vi "Autonomous Independent.vi"() -> ()   [LabVIEW 2012]
doc: "This VI is called when autonomous begins, and will automatically be terminated when autonomous ends. You can carry out timed or sensor driven robot movement independently without needing to return to the caller."
uses:
  <vilib>/Rock Robotics/WPI/SafetyOutput/WPI_SafetyOutputConfigMenu.ctl
  Robot Global Data.vi
  Autonomous Global Data.vi
  <vilib>/Rock Robotics/WPI/RobotDrive/WPI_RobotDriveGetSetRefNum.vi
  <vilib>/Rock Robotics/WPI/RobotDrive/WPI_RobotDriveMecanumDrive_Cartesian.vi
  <vilib>/Rock Robotics/WPI/Joystick/WPI_JoystickGetSetRefNum.vi
  <vilib>/Rock Robotics/WPI/RobotDrive/WPI_RobotDriveArcadeDrive.vi
panel:
  in  "time":dbl
  in  "File Name With Extension 3":string="test1.cat"
  in  "File Name With Extension 2":string="test1.cat"
  in  "File Name With Extension 1":string="test1.cat"
  out "Autonomous Mode":u16(ring) items=["None", "Scripted", "Hybrided"]
  out "error out":errorcluster
  in  "File Name With Extension 0":string="test1.cat"
  out "File Status":string
  out "Lines":string[](array[string])
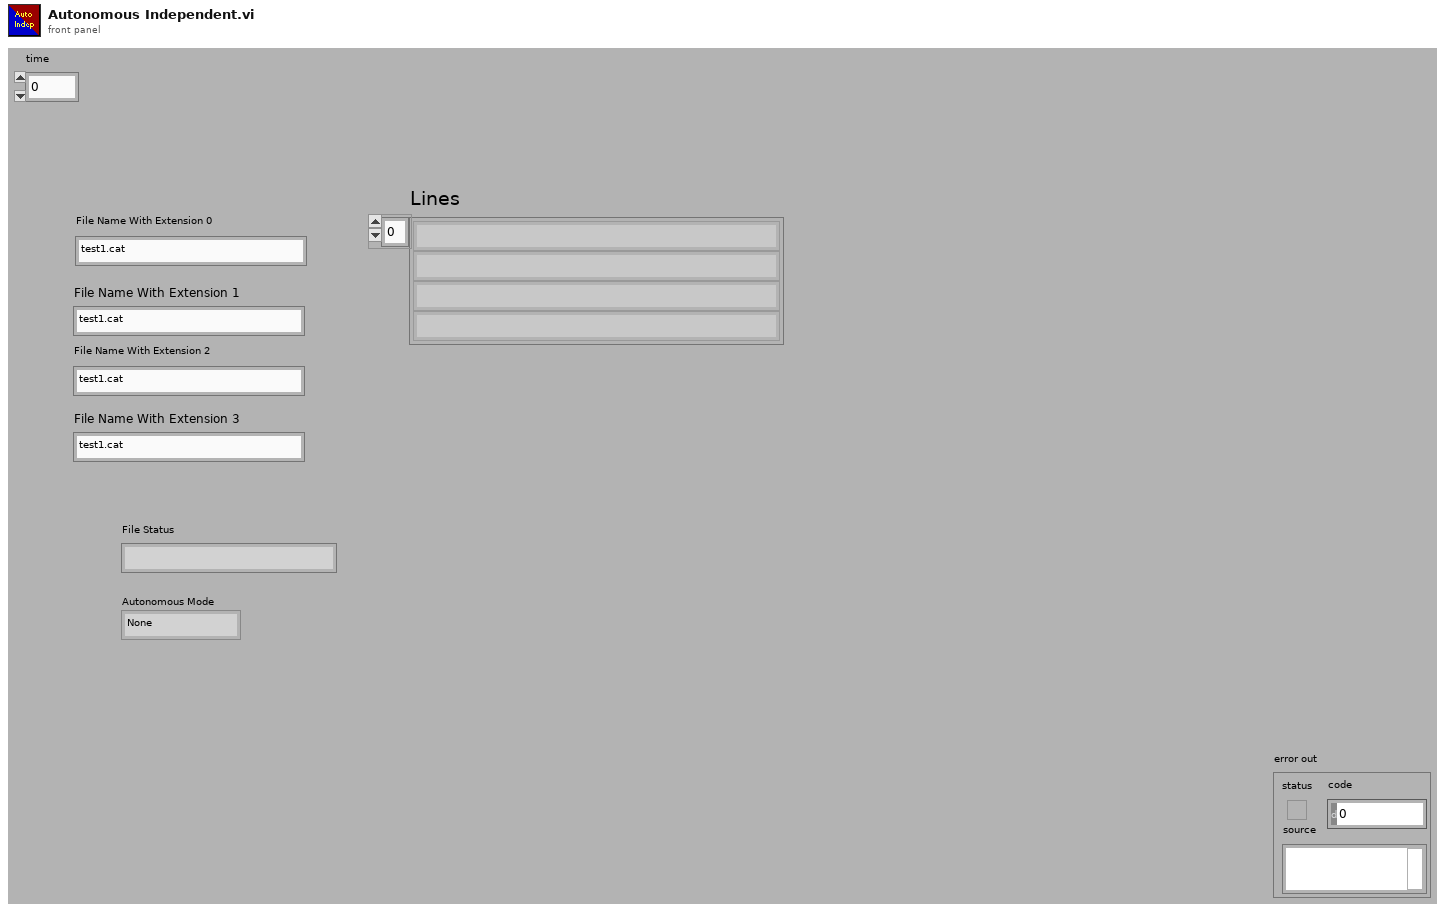
[diagram p1: front panel]
types:
  T1 = typedef "WPI_JoystickDevRef.ctl" = cluster{"Device":T2}
  T2 = typedef "WPI_JoystickDeviceEnum.ctl" = enum16{"USB 1", "USB 2", "USB 3", "USB 4", "Kinect 1", "Kinect 2"}
  T3 = cluster{"axis 1 (x)":dbl, "axis 2 (y)":dbl, "axis 3 (throttle)":dbl, "axis 4":dbl, "axis 5":dbl, "axis 6":dbl}
  T4 = typedef "WPI_SafetyOutputConfigMenu.ctl" = enum16{"Enable", "Disable"}
  T5 = typedef "WPI_RobotDriveDevRef.ctl" = cluster{"DevStatus":errorcluster, "Motors[]":T6[], "Square Inputs":bool, "Max Output":dbl, "Isochronous":bool}
  T6 = typedef "WPI_MotorControlDeviceRef.ctl" = cluster{"DeviceStatus":errorcluster, "Type":enum16{"PWM", "CAN"}, "PWM":cluster{"Digital Module":T7, "PWM Channel":T8, "DeadBand":T9}, "CAN":cluster{"Device Number":u8, "Control Mode":T10, "Semaphore":T11, "Max Vout":dbl}, "Invert":bool, "TransformRef":T12, "InvTransformRef":T12}
  T7 = typedef "FPGA_TypedefDigitalModule.ctl" = enum16{"Digital Module 1", "Digital Module 2"}
  T8 = typedef "FPGA_DIOPWMChannel.ctl" = enum8{"PWM 1", "PWM 2", "PWM 3", "PWM 4", "PWM 5", "PWM 6", "PWM 7", "PWM 8", "PWM 9", "PWM 10", "Invalid"}
  T9 = typedef "WPI_PWMDeadband.ctl" = cluster{"Name":string, "maxPositivePwm":i32, "minPositivePwm":i32, "centerPwm":i32, "maxNegativePwm":i32, "minNegativePwm":i32, "angularRange":u16}
  T10 = typedef "WPI_CANJaguar_ControlMode.ctl" = enum8{"Percent VBus", "Current", "Speed", "Position", "Voltage"}
  T11 = typedef "Semaphore RefNum" = refnum<k1>
  T12 = typedef "WPI_PWMTransform_ConPane.ctl" = refnum<vi>
  T13 = cluster{"RightAxis":dbl, "LeftAxis":dbl, "RightHead":bool, "Left Head":bool, "Left Leg Out":bool, "Left Leg Forward":bool, "Left Leg Back":bool, "Right Leg Out":bool, "Right Leg Forward":bool, "Right Leg Back":bool}
  T14 = cluster{"Position":cluster{"X":dbl, "Y":dbl}, "Distance (ft)":dbl}[]
  T15 = cluster{"Position":cluster{"X":dbl, "Y":dbl}, "Distance (ft)":dbl}
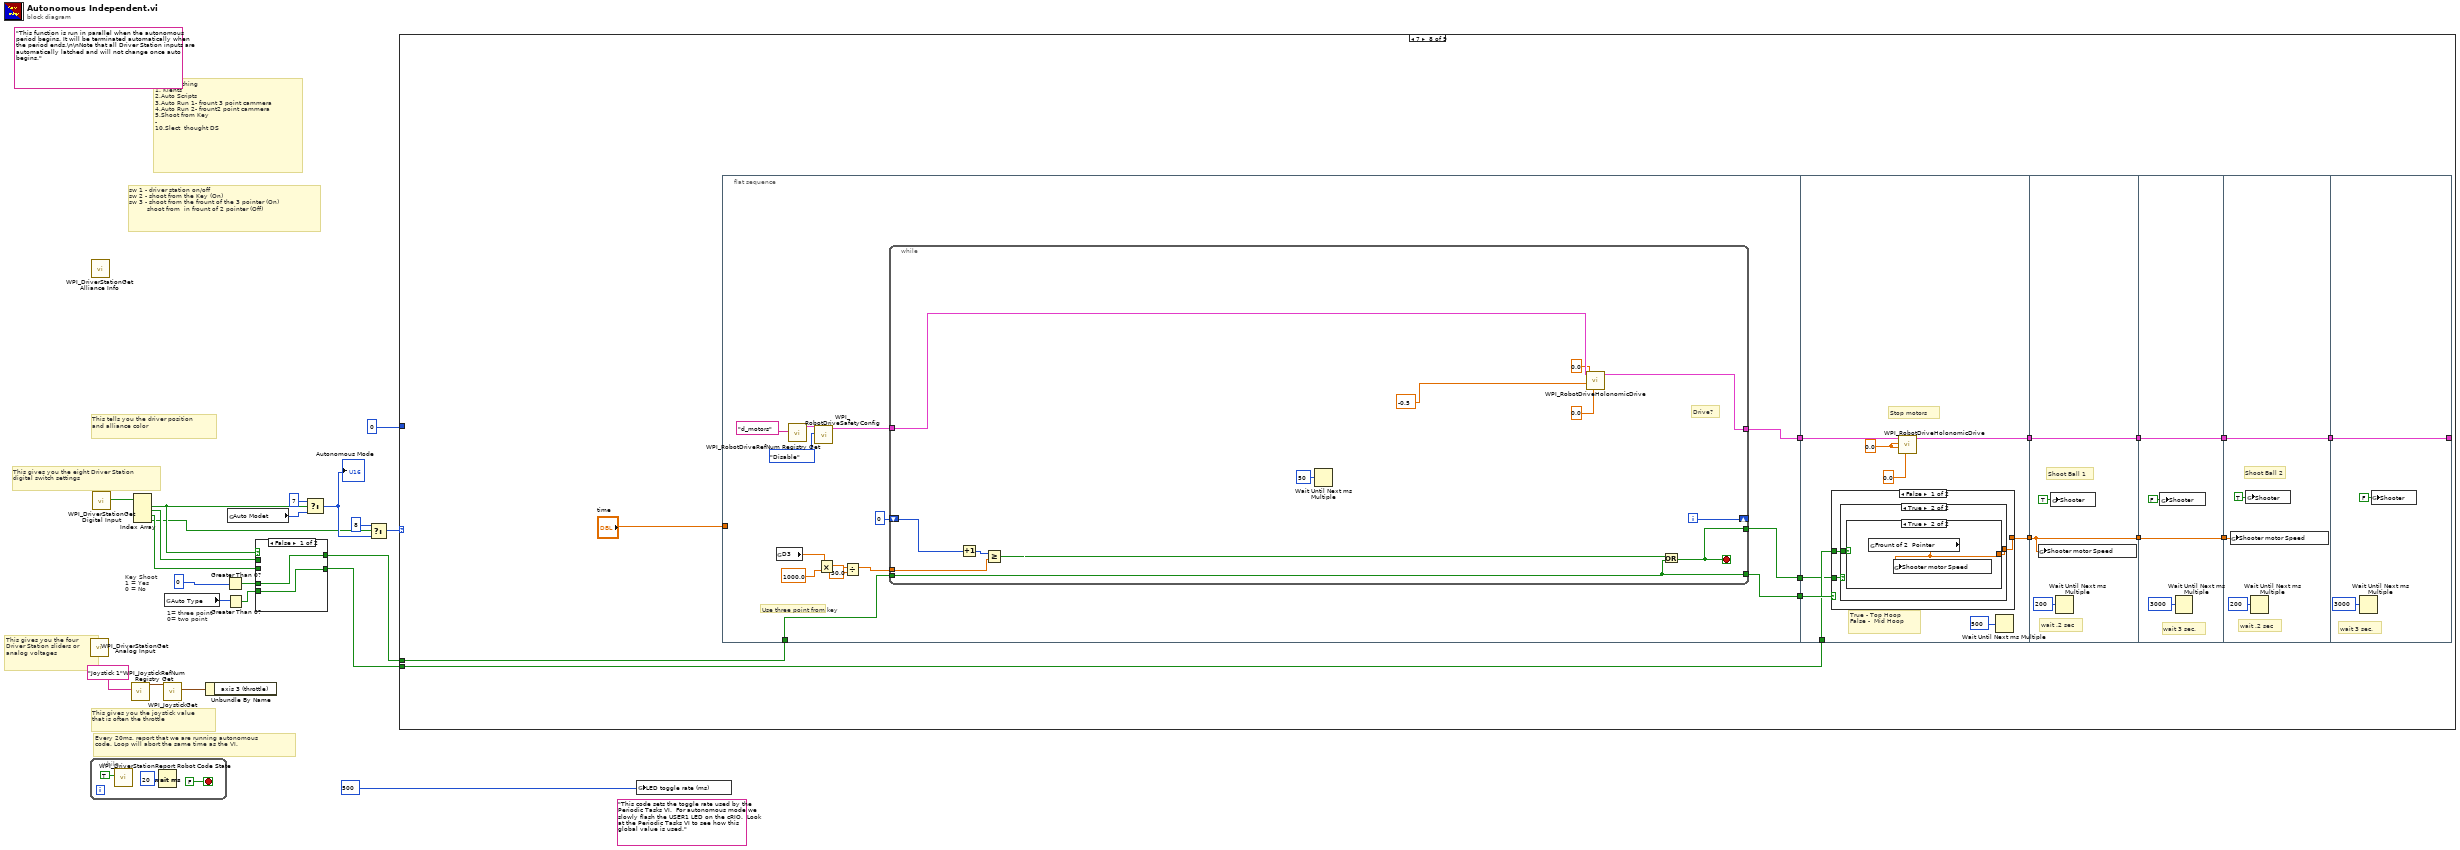
[diagram p0: block diagram]
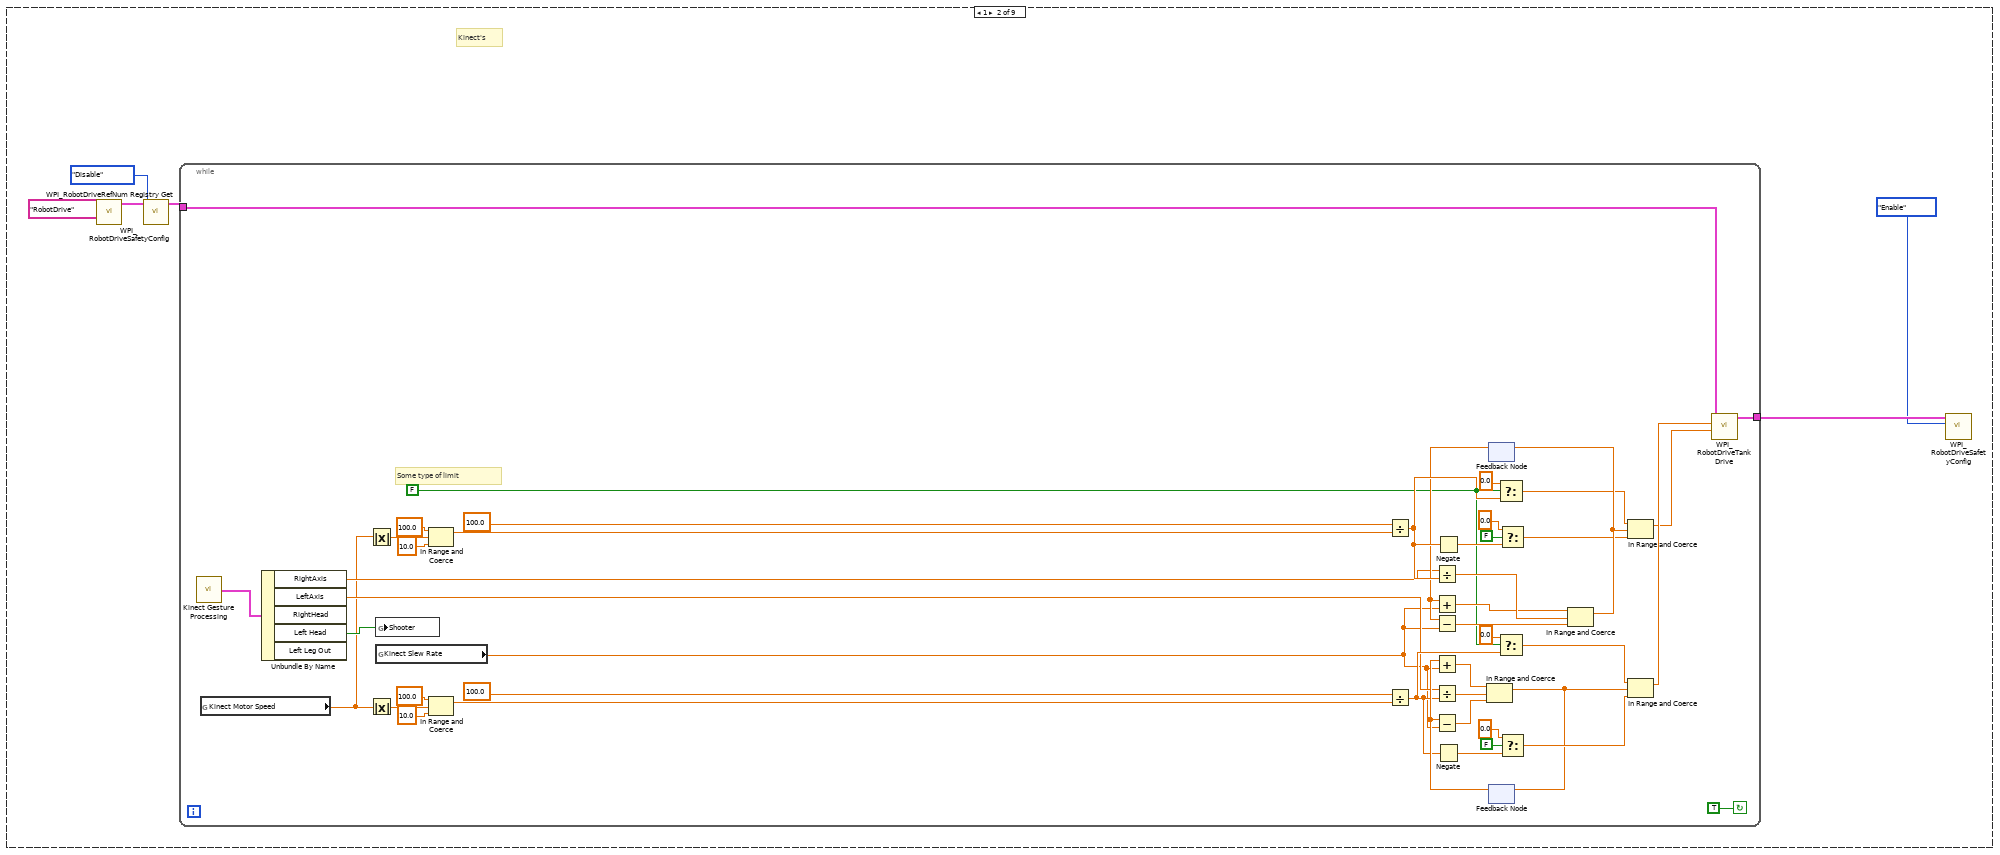
[diagram p4: hidden frame]
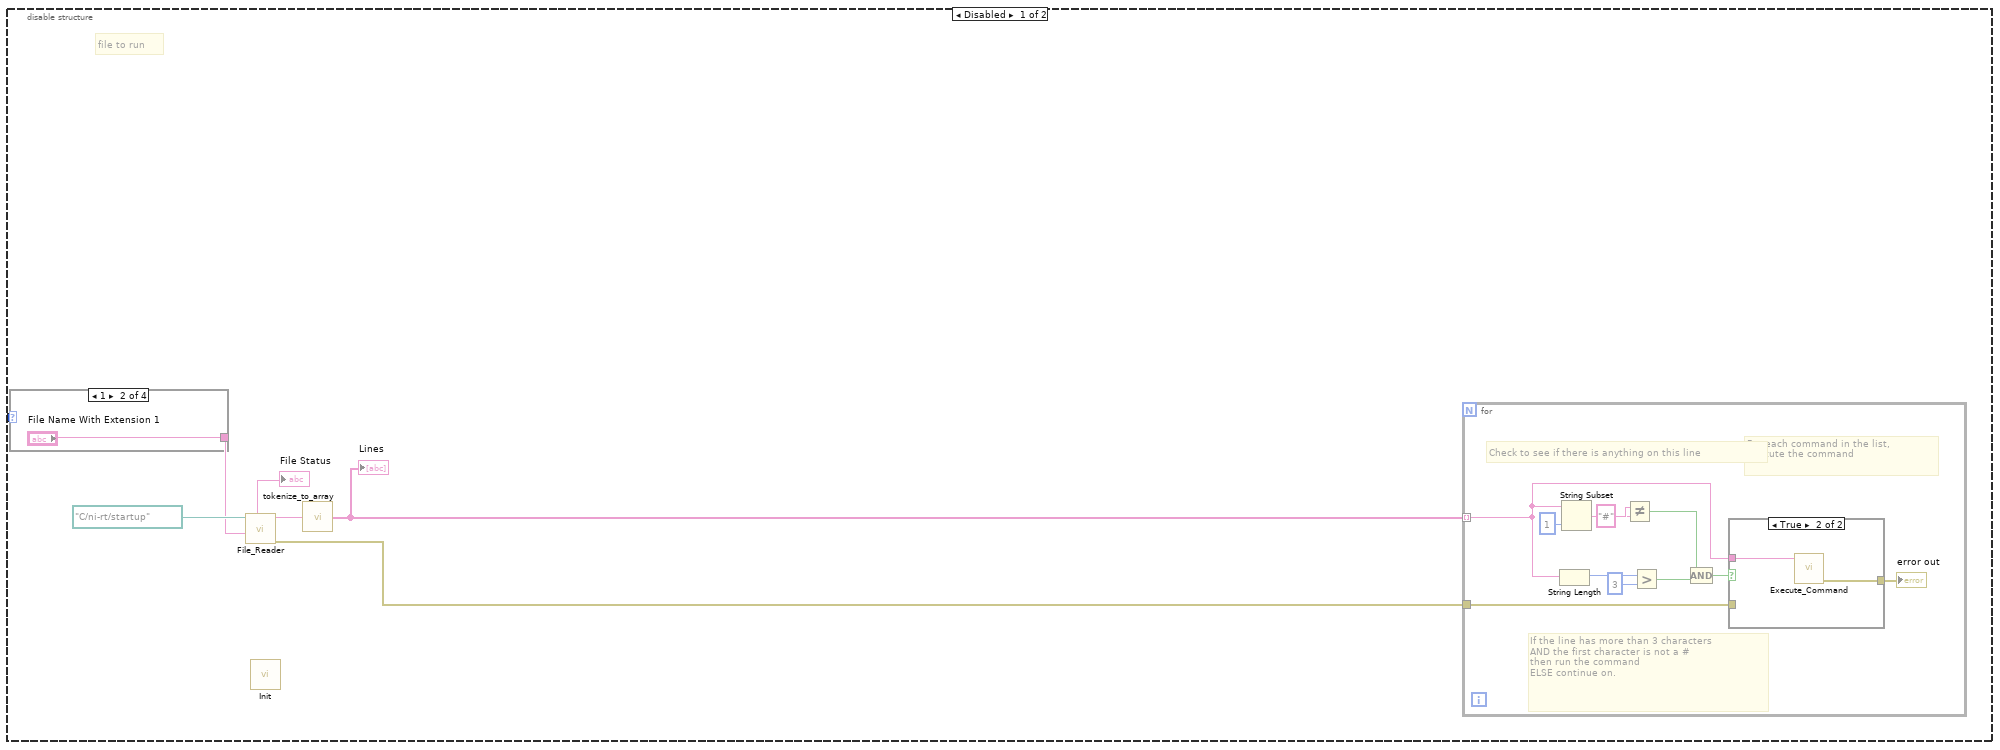
[diagram p6: hidden frame]
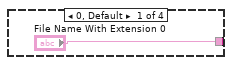
[diagram p7: hidden frame]
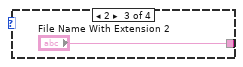
[diagram p8: hidden frame]
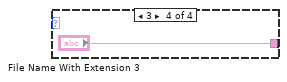
[diagram p9: hidden frame]
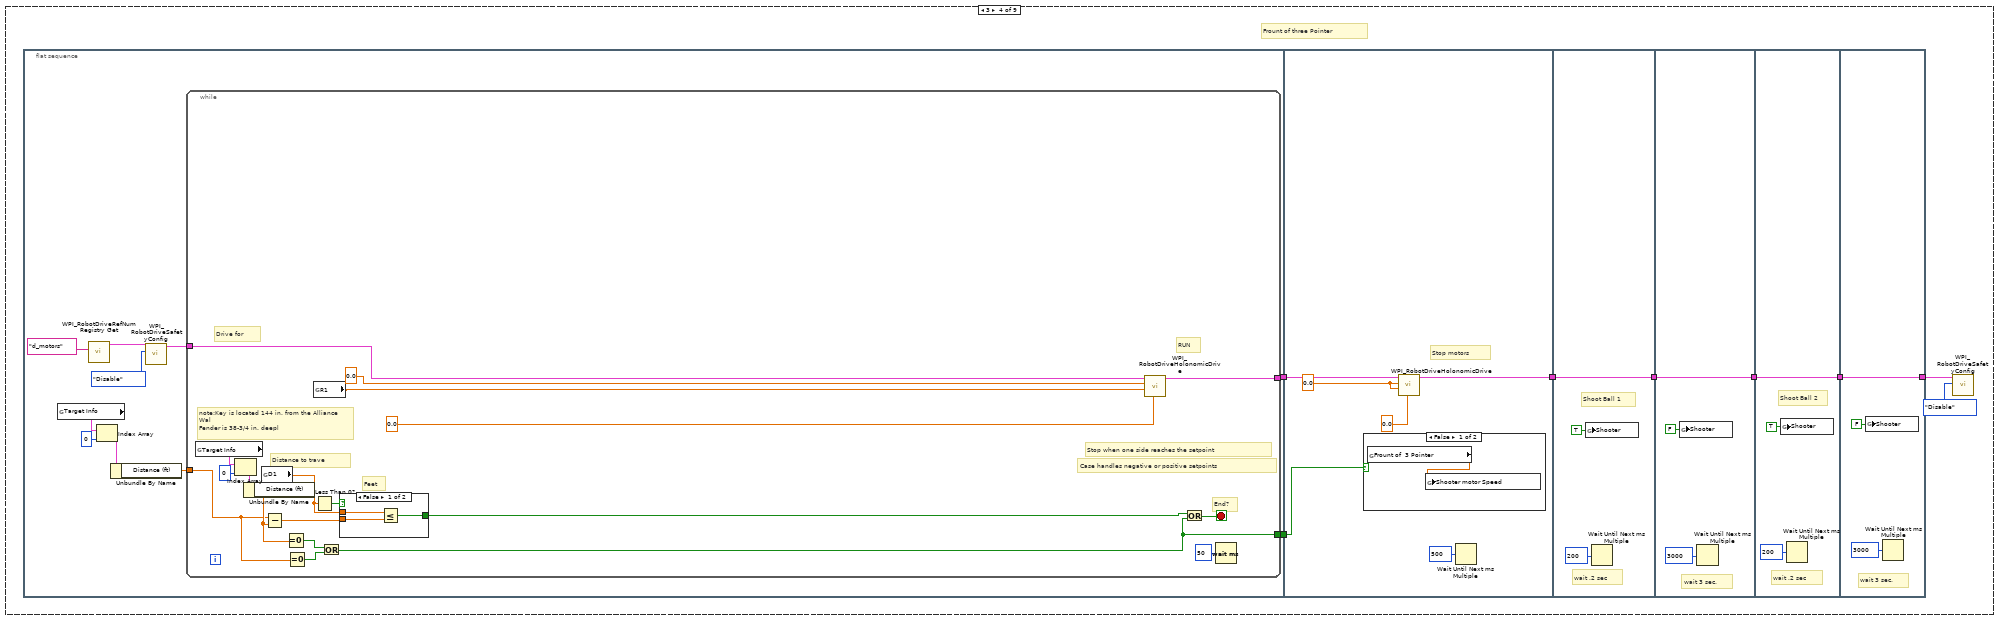
[diagram p11: hidden frame]
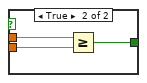
[diagram p12: hidden frame]
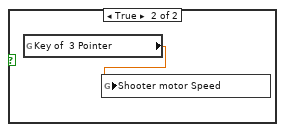
[diagram p13: hidden frame]
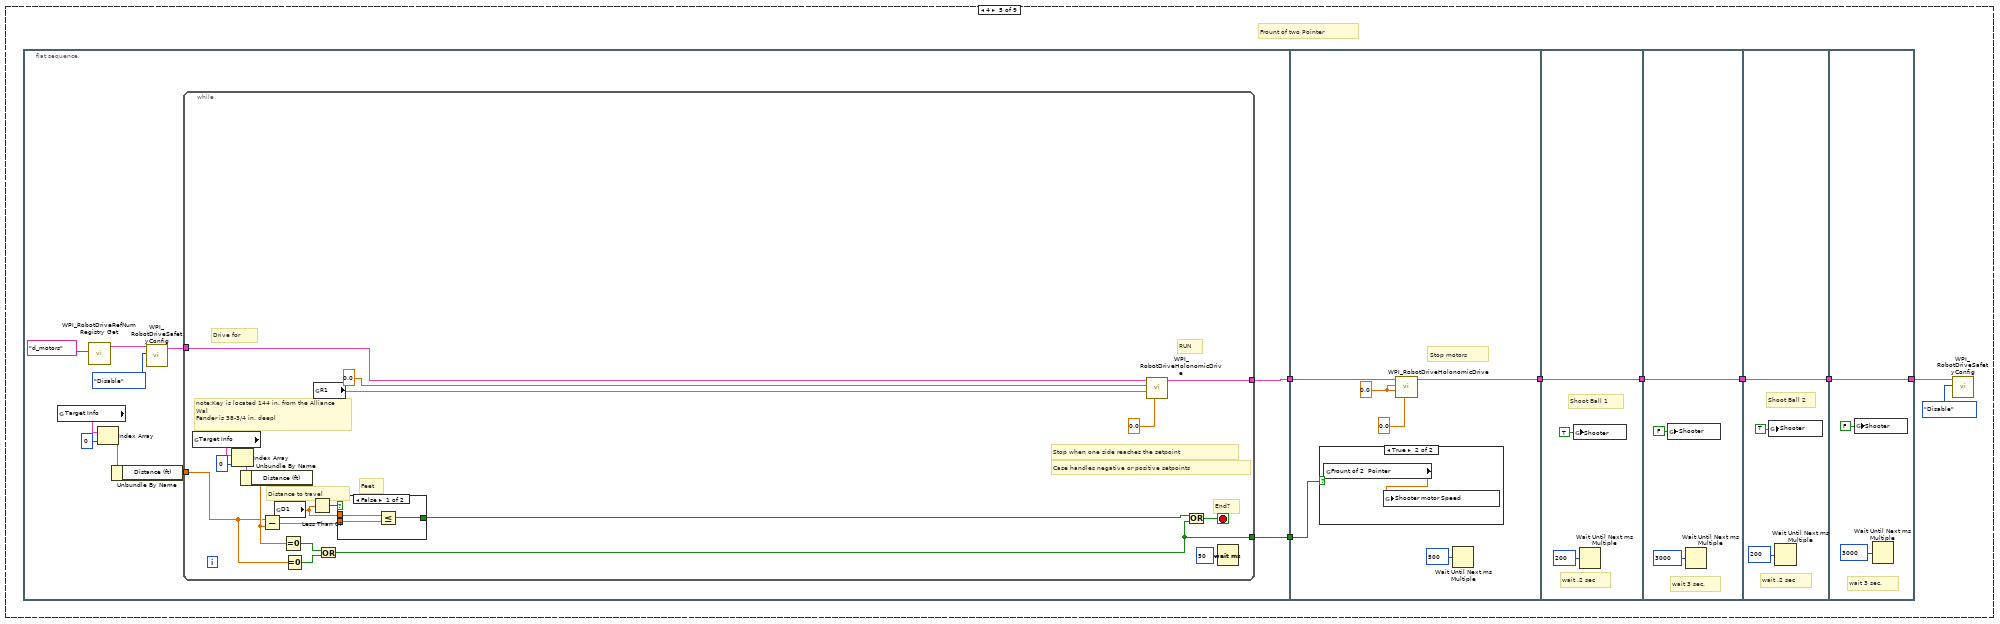
[diagram p14: hidden frame]
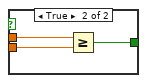
[diagram p15: hidden frame]
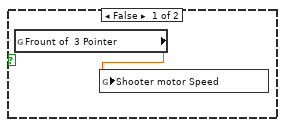
[diagram p16: hidden frame]
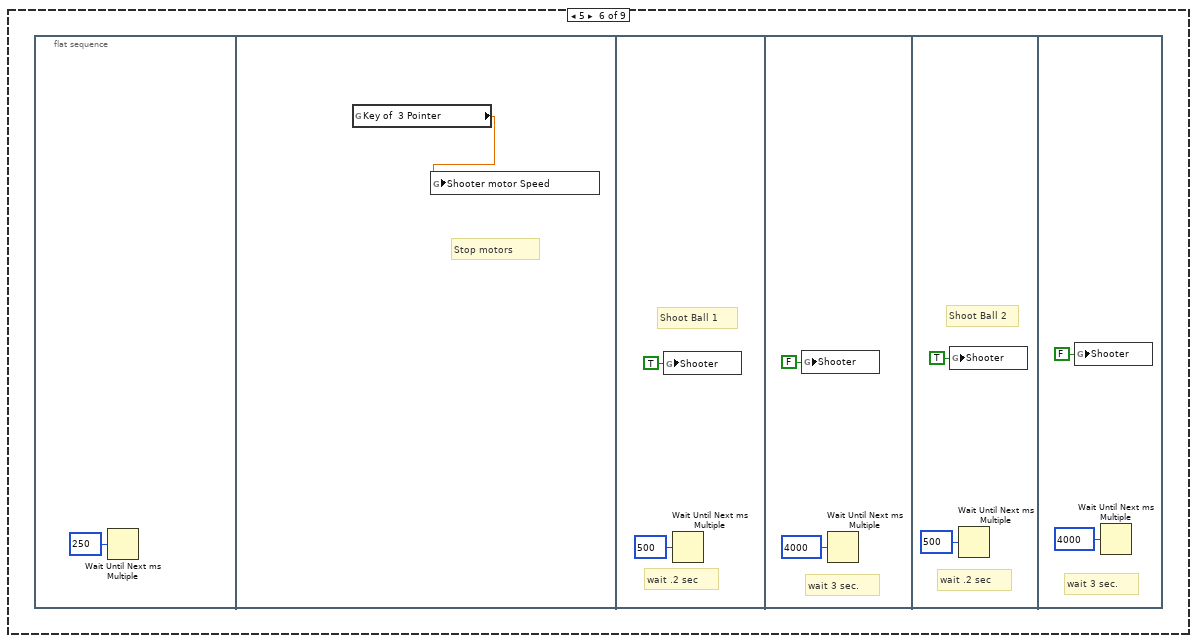
[diagram p17: hidden frame]
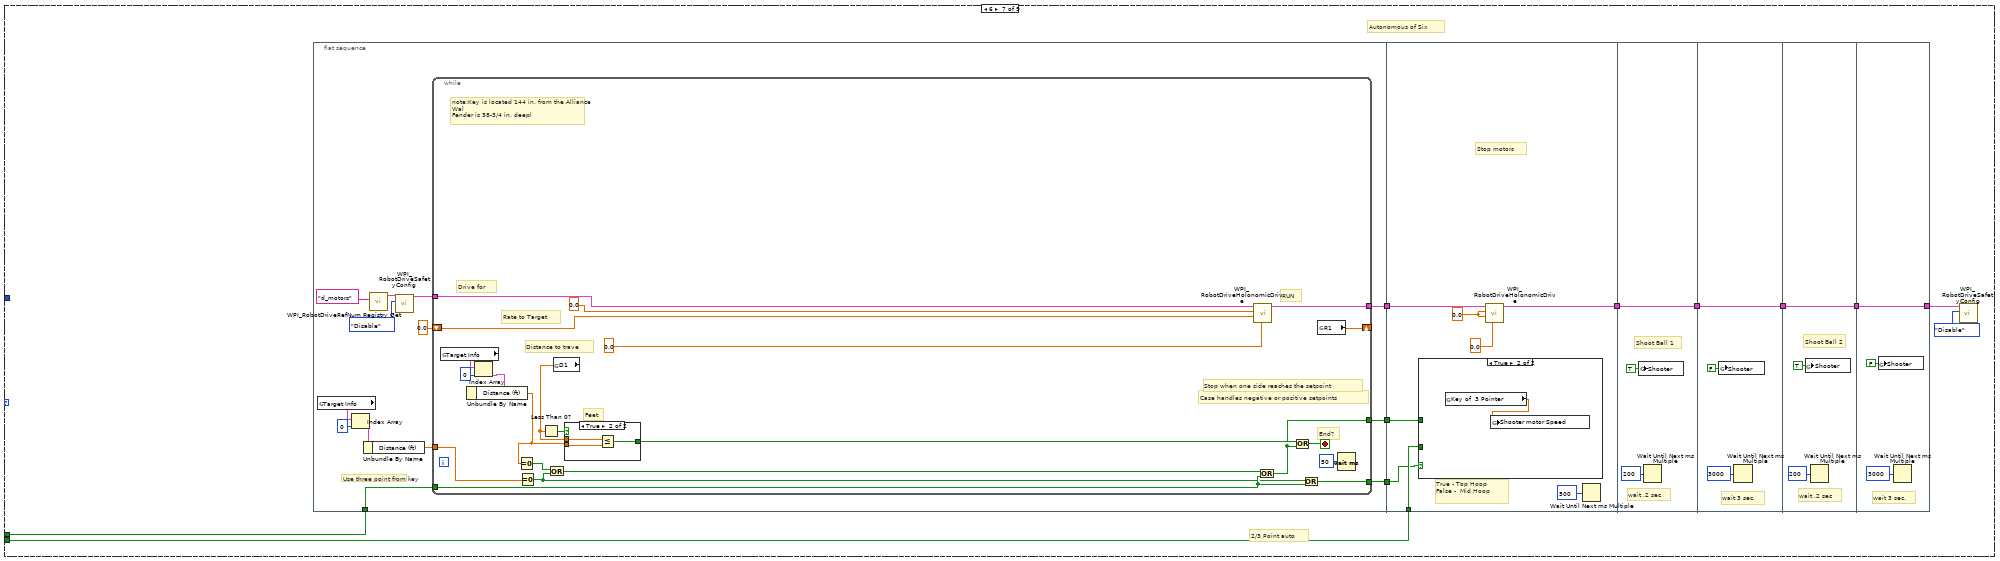
[diagram p18: hidden frame]
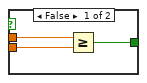
[diagram p19: hidden frame]
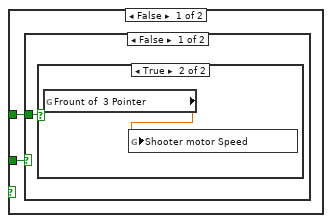
[diagram p20: hidden frame]
diagram:
  (unwired) "This code sets the toggle rate used by the Periodic Tasks VI.  For autonomous mode we slowly flash the USER1 LED on the cRIO.  Look at the Periodic Tasks VI to see how this global value is used."
  (unwired) "This function is run in parallel when the autonomous period begins. It will be terminated automatically when the period ends.\n\nNote that all Driver Station inputs are automatically latched and will not change once auto begins."
  # "Key Shoot\n1 = Yes\n0 = No"
  # "sw 1 - driver station on/off\nsw 2 - shoot from the Key (On)\nsw 3 - shoot from the frount of the 3 pointer (On)\n         shoot from  in frount of 2 pointer (Off)"
  # "1= three point\n0= two point"
  # "0. Do nothing\n1. Kients\n2.Auto Scripts\n3.Auto Run 1- frount 3 point cammera\n4.Auto Run 2- frount2 point cammera\n5.Shoot from Key\n-\n10.Slect  thought DS"
  # "Every 20ms, report that we are running autonomous\ncode. Loop will abort the same time as the VI."
  # "This gives you the joystick value\nthat is often the throttle"
  # "This tells you the driver position\nand alliance color"
  # "This gives you the eight Driver Station\ndigital switch settings"
  # "This gives you the four\nDriver Station sliders or\nanalog voltages"
  n1 = call <vilib>:"WPI_DriverStationGet Analog Input.vi"() -> ()  [unwired: 12 out]
  n2 = while {
    stop <- FALSE stop-if-true
    n3 = call <vilib>:"WPI_DriverStationReport Robot Code State.vi"("Autonomous"=TRUE) -> ()  [unwired: 10 in, 1 out]
    n4 = Wait (ms)(milliseconds to wait=u32 20) -> ()  [unwired: 1 out]
  }
  n5 = call <vilib>:"WPI_DriverStationGet Alliance Info.vi"() -> ()  [unwired: 12 out]
  n6 = call <vilib>:"WPI_DriverStationGet Digital Input.vi"() -> ("Driver Station Digital Input (1-8)"=w21:bool[])  [unwired: 11 out]
  n7 = call <vilib>:"WPI_JoystickRefNum Registry Get.vi"("refnum name"="Joystick 1") -> ("JoystickDevRef"=w18:T1)  [unwired: 1 in, 9 out]
  n8 = Index Array(array=w21) -> (element #1=w8:bool, element #2=w7:bool, element #3=w6:bool, element #4=w4:bool)  [unwired: 4 in]
  n9 = call <vilib>:"WPI_JoystickGet.vi"("JoystickDevRef"=w18) -> ("Axes"=w19:T3)  [unwired: 1 in, 5 out]
  n10 = global read "Autonomous Global Data.vi" "Auto Type"() -> (w14:u16)
  n11 = Unbundle By Name(w19) -> ()  [unwired: 1 out]
  n12 = Greater Than 0?(x=u16 0 ("t")) -> (x > 0?=w13:bool)
  n13 = Greater Than 0?(x=w14) -> (x > 0?=w12:bool)
  n14 = global read "Autonomous Global Data.vi" "Auto Modet"() -> (w10:u16)
  n15 = case shown="False" w8 {
    tunnel: w7 -> [_ w28]
    tunnel: w6 -> [_ w27]
    tunnel: [w26 w28] -> w16
    tunnel: [w25 w27] -> w15
    tunnel: w13 -> [w26 _]
    tunnel: w12 -> [w25 _]
    frame False {
    }
    frame True {
    }
  }
  n16 = Select(t=u16 7, s=w8, f=w10) -> (s? t:f=w11:u16)
  "Autonomous Mode" <- w11
  n17 = Select(t=u16 8, s=w4, f=w11) -> (s? t:f=w5:u16)
  n18 = case shown="7" w5 {
    tunnel: 0 -> [_ _ w81 _ _ _ _ _ _]
    tunnel: w15 -> [_ _ _ _ _ _ w245 w330 _]
    tunnel: w16 -> [_ _ _ _ _ _ w244 w331 _]
    frame 0, Default {
      # "Do nothing"
    }
    frame 1 {
      # "Kinect's"
      n19 = call <vilib>:"WPI_RobotDriveRefNum Registry Get.vi"("refnum name"="RobotDrive") -> ("RobotDriveDevRef"=w33:T5)  [unwired: 9 in, 1 out]
      n20 = call <vilib>:"WPI_RobotDriveSafetyConfig.vi"("mode"=WPI_SafetyOutputConfigMenu."Disable", "RobotDriveDevRef"=w33) -> ("RobotDriveDevRef"=w32:T5)  [unwired: 8 in, 1 out]
      n21 = while {
        tunnel: w32 -> [w79]
        tunnel: [w35] -> w30
        stop <- TRUE continue-if-true
        w36 = FALSE
        # "Some type of limit"
        n22 = call "Kinect Gesture Processing.vi"() -> ("Joystick Data"=w80:T13)  [unwired: 1 in]
        n23 = global read "Robot Global Data.vi" "Kinect Motor Speed"() -> (w40:dbl)
        n24 = Unbundle By Name(w80) -> ("RightAxis"=w42:dbl, "LeftAxis"=w41:dbl, "Left Head"=w77:bool)  [unwired: 2 out]
        n25 = Absolute Value(x=w40) -> (abs(x)=w50:dbl)
        n26 = Absolute Value(x=w40) -> (abs(x)=w67:dbl)
        n27 = global write "Robot Global Data.vi" "Shooter"(w77) -> ()
        n28 = global read "Robot Global Data.vi" "Kinect Slew Rate"() -> (w39:dbl)
        n29 = In Range and Coerce(upper limit=100.0, x=w50, lower limit=10.0) -> (coerced(x)=w53:dbl)  [unwired: 1 out]
        n30 = In Range and Coerce(upper limit=100.0, x=w67, lower limit=10.0) -> (coerced(x)=w64:dbl)  [unwired: 1 out]
        n31 = Divide(x=100.0, y=w53) -> (x/y=w56:dbl)
        n32 = Divide(x=100.0, y=w64) -> (x/y=w61:dbl)
        n33 = Divide(x=w42, y=w56) -> (x/y=w54:dbl)
        n34 = Divide(x=w41, y=w61) -> (x/y=w63:dbl)
        n35 = Negate(x=w56) -> (-x=w57:dbl)
        n36 = Negate(x=w61) -> (-x=w60:dbl)
        n37 = feedback #1() -> (w47:dbl)  [unwired: 1 in]
        n38 = Add(x=w47, y=w39) -> (x+y=w49:dbl)
        n39 = Subtract(x=w47, y=w39) -> (x-y=w48:dbl)
        n40 = feedback #2() -> (w70:dbl)  [unwired: 1 in]
        n41 = Add(x=w70, y=w39) -> (x+y=w68:dbl)
        n42 = Subtract(x=w70, y=w39) -> (x-y=w69:dbl)
        n43 = In Range and Coerce(upper limit=w68, x=w63, lower limit=w69) -> (coerced(x)=w62:dbl)  [unwired: 1 out]
        n44 = feedback-in #2(w62) -> ()
        n45 = Select(t=0.0, s=w36, f=w56) -> (s? t:f=w43:dbl)
        n46 = Select(t=0.0, s=w36, f=w61) -> (s? t:f=w74:dbl)
        n47 = Select(t=0.0, s=FALSE, f=w57) -> (s? t:f=w44:dbl)
        n48 = Select(t=0.0, s=FALSE, f=w60) -> (s? t:f=w73:dbl)
        n49 = In Range and Coerce(upper limit=w49, x=w54, lower limit=w48) -> (coerced(x)=w55:dbl)  [unwired: 1 out]
        n50 = feedback-in #1(w55) -> ()
        n51 = In Range and Coerce(upper limit=w43, x=w55, lower limit=w44) -> (coerced(x)=w37:dbl)  [unwired: 1 out]
        n52 = In Range and Coerce(upper limit=w74, x=w62, lower limit=w73) -> (coerced(x)=w38:dbl)  [unwired: 1 out]
        n53 = call <vilib>:"WPI_RobotDriveTankDrive.vi"("Right axis value"=w37, "Left axis value"=w38, "RobotDriveDevRef"=w79) -> ("RobotDriveDevRef"=w35:T5)  [unwired: 6 in, 2 out]
      }
      n54 = call <vilib>:"WPI_RobotDriveSafetyConfig.vi"("mode"=WPI_SafetyOutputConfigMenu."Enable", "RobotDriveDevRef"=w30) -> ()  [unwired: 8 in, 2 out]
    }
    frame 2 {
      n55 = disable-structure shown="Enabled" {
        disable-tunnel: w81 -> [w85 _]
        frame Disabled {
          # "file to run"
          n56 = case shown="1" w85 {
            tunnel: ["File Name With Extension 0" "File Name With Extension 1" "File Name With Extension 2" "File Name With Extension 3"] -> w82
            frame 0, Default {
            }
            frame 1 {
            }
            frame 2 {
            }
            frame 3 {
            }
          }
          n57 = call "File_Reader.vi"("File Name With Extension"=w82, "Path"=path "C:/ni-rt/startup") -> ("error out"=w86:errorcluster, "File Contents"=w88:string, "File status"=→"File Status":string)  [unwired: 2 in, 3 out]
          n58 = call "Init.vi"() -> ()  [unwired: 12 in]
          n59 = call "tokenize_to_array.vi"("File Contents"=w88) -> ("Lines"=w87:string[])
          "Lines" <- w87
          n60 = for {
            tunnel: w86 -> [w94]
            tunnel: w87 -> [w93] mode=indexing
            # "If the line has more than 3 characters\nAND the first character is not a #\nthen run the command\nELSE continue on."
            # "Check to see if there is anything on this line"
            # "For each command in the list,\nexecute the command"
            n61 = String Length(string=w93) -> (length=w103:i32)
            n62 = String Subset(string=w93, length (rest)=1 ("length (rest)")) -> (substring=w98:string)  [unwired: 1 out]
            n63 = Not Equal?(x=w98, y="#") -> (x != y?=w96:bool)
            n64 = Greater?(x=w103, y=3) -> (0:w100:bool)
            n65 = Compound Arithmetic op=AND(w96, w100) -> (w101:bool)
            n66 = case shown="True" w101 {
              tunnel: w93 -> [_ w106]
              tunnel: [w104 w105] -> w95
              tunnel: w94 -> [w104 _]
              frame False {
              }
              frame True {
                n67 = call "Execute_Command.vi"("Command"=w106) -> ("error out"=w105:errorcluster)  [unwired: 8 in, 2 out]
              }
            }
            "error out" <- w95
          }
        }
        frame Enabled {
        }
      }
    }
    frame 3 {
      # "Frount of three Pointer"
      n68 = flat-sequence {
        tunnel: [w120] -> w114
        tunnel: [w119] -> w113
        tunnel: w114 -> [w153]
        tunnel: w113 -> [w151]
        tunnel: [w150] -> w111
        tunnel: [w158] -> w112
        tunnel: w111 -> [w158]
        tunnel: w112 -> [w161]
        tunnel: [w161] -> w109
        tunnel: [w164] -> w110
        tunnel: w109 -> [w164]
        tunnel: w110 -> [w167]
        tunnel: [w167] -> w108
        frame #0 {
          n69 = global read "Robot Global Data.vi" "Target Info"() -> (w123:T14)
          n70 = call <vilib>:"WPI_RobotDriveRefNum Registry Get.vi"("refnum name"="d_motors") -> ("RobotDriveDevRef"=w117:T5)  [unwired: 1 in, 9 out]
          n71 = Index Array(array=w123, index=0) -> (element=w122:T15)
          n72 = Unbundle By Name(w122) -> ("Distance (ft)"=w121:dbl)
          n73 = call <vilib>:"WPI_RobotDriveSafetyConfig.vi"("mode"=WPI_SafetyOutputConfigMenu."Disable", "RobotDriveDevRef"=w117) -> ("RobotDriveDevRef"=w115:T5)  [unwired: 8 in, 1 out]
          n74 = while {
            tunnel: w121 -> [w133]
            tunnel: [w139] -> w120
            tunnel: [w129] -> w119
            tunnel: w115 -> [w127]
            stop <- w130 stop-if-true
            # "Distance to trave"
            # "note:Key is located 144 in. from the Alliance Wal\nFender is 38-3/4 in. deepl"
            # "Drive for"
            # "Feet"
            # "RUN"
            # "Case handles negative or positive setpoints"
            # "End?"
            # "Stop when one side reaches the setpoint"
            n75 = global read "Robot Global Data.vi" "Target Info"() -> (w128:T14)
            n76 = Index Array(array=w128, index=0) -> (element=w138:T15)
            n77 = Unbundle By Name(w138) -> ("Distance (ft)"=w134:dbl)
            n78 = global read "Autonomous Global Data.vi" "D1"() -> (w125:dbl)
            n79 = Subtract(x=w133, y=w134) -> (x-y=w136:dbl)
            n80 = Equal To 0?(x=w134) -> (x = 0?=w132:bool)
            n81 = Equal To 0?(x=w133) -> (x = 0?=w131:bool)
            n82 = global read "Autonomous Global Data.vi" "R1"() -> (w126:dbl)
            n83 = Less Than 0?(x=w125) -> (x < 0?=w142:bool)
            n84 = Or(x=w132, y=w131) -> (x .or. y?=w129:bool)
            n85 = case shown="False" w142 {
              tunnel: w125 -> [w146 w149]
              tunnel: w136 -> [w145 w148]
              tunnel: [w144 w147] -> w135
              frame False {
                n86 = Less Or Equal?(x=w146, y=w145) -> (x <= y?=w144:bool)
              }
              frame True {
                n87 = Greater Or Equal?(x=w149, y=w148) -> (x >= y?=w147:bool)
              }
            }
            n88 = call-poly <vilib>:"WPI_RobotDriveHolonomicDrive.vi"("Rotation"=0.0, "Y"=w126, "X"=0.0, "RobotDriveDevRef"=w127) -> ("RobotDriveDevRef"=w139:T5)  [unwired: 5 in, 2 out]
            n89 = Or(x=w135, y=w129) -> (x .or. y?=w130:bool)
            n90 = Wait (ms)(milliseconds to wait=u32 50) -> ()  [unwired: 1 out]
          }
        }
        frame #1 {
          w154 = 0.0 ("X")
          # "Stop motors"
          n91 = case shown="False" w151 {
            frame False {
              n92 = global read "Robot Global Data.vi" "Frount of  3 Pointer"() -> (w156:dbl)
              n93 = global write "Robot Global Data.vi" "Shooter motor Speed"(w156) -> ()
            }
            frame True {
              n94 = global read "Robot Global Data.vi" "Key of  3 Pointer"() -> (w157:dbl)
              n95 = global write "Robot Global Data.vi" "Shooter motor Speed"(w157) -> ()
            }
          }
          n96 = call-poly <vilib>:"WPI_RobotDriveHolonomicDrive.vi"("Rotation"=0.0, "Y"=w154, "X"=w154, "RobotDriveDevRef"=w153) -> ("RobotDriveDevRef"=w150:T5)  [unwired: 5 in, 2 out]
          n97 = Wait Until Next ms Multiple(millisecond multiple=u32 500) -> ()  [unwired: 1 out]
        }
        frame #2 {
          # "Shoot Ball 1"
          # "wait .2 sec"
          n98 = global write "Robot Global Data.vi" "Shooter"(TRUE ("Shooter")) -> ()
          n99 = Wait Until Next ms Multiple(millisecond multiple=u32 200) -> ()  [unwired: 1 out]
        }
        frame #3 {
          # "wait 3 sec."
          n100 = global write "Robot Global Data.vi" "Shooter"(FALSE ("Shooter")) -> ()
          n101 = Wait Until Next ms Multiple(millisecond multiple=u32 3000) -> ()  [unwired: 1 out]
        }
        frame #4 {
          # "Shoot Ball 2"
          # "wait .2 sec"
          n102 = global write "Robot Global Data.vi" "Shooter"(TRUE ("Shooter")) -> ()
          n103 = Wait Until Next ms Multiple(millisecond multiple=u32 200) -> ()  [unwired: 1 out]
        }
        frame #5 {
          # "wait 3 sec."
          n104 = global write "Robot Global Data.vi" "Shooter"(FALSE ("Shooter")) -> ()
          n105 = Wait Until Next ms Multiple(millisecond multiple=u32 3000) -> ()  [unwired: 1 out]
        }
      }
      n106 = call <vilib>:"WPI_RobotDriveSafetyConfig.vi"("mode"=WPI_SafetyOutputConfigMenu."Disable", "RobotDriveDevRef"=w108) -> ()  [unwired: 8 in, 2 out]
    }
    frame 4 {
      # "Frount of two Pointer"
      n107 = flat-sequence {
        tunnel: [w183] -> w177
        tunnel: [w182] -> w176
        tunnel: w177 -> [w216]
        tunnel: w176 -> [w213]
        tunnel: [w214] -> w174
        tunnel: [w221] -> w175
        tunnel: w174 -> [w221]
        tunnel: w175 -> [w224]
        tunnel: [w224] -> w172
        tunnel: [w227] -> w173
        tunnel: w172 -> [w227]
        tunnel: w173 -> [w230]
        tunnel: [w230] -> w171
        frame #0 {
          n108 = global read "Robot Global Data.vi" "Target Info"() -> (w186:T14)
          n109 = call <vilib>:"WPI_RobotDriveRefNum Registry Get.vi"("refnum name"="d_motors") -> ("RobotDriveDevRef"=w180:T5)  [unwired: 1 in, 9 out]
          n110 = Index Array(array=w186, index=0) -> (element=w185:T15)
          n111 = Unbundle By Name(w185) -> ("Distance (ft)"=w184:dbl)
          n112 = call <vilib>:"WPI_RobotDriveSafetyConfig.vi"("mode"=WPI_SafetyOutputConfigMenu."Disable", "RobotDriveDevRef"=w180) -> ("RobotDriveDevRef"=w178:T5)  [unwired: 8 in, 1 out]
          n113 = while {
            tunnel: w184 -> [w196]
            tunnel: [w202] -> w183
            tunnel: [w192] -> w182
            tunnel: w178 -> [w190]
            stop <- w193 stop-if-true
            # "Distance to travel"
            # "note:Key is located 144 in. from the Alliance Wal\nFender is 38-3/4 in. deepl"
            # "Drive for"
            # "Feet"
            # "RUN"
            # "Case handles negative or positive setpoints"
            # "End?"
            # "Stop when one side reaches the setpoint"
            n114 = global read "Robot Global Data.vi" "Target Info"() -> (w191:T14)
            n115 = Index Array(array=w191, index=0) -> (element=w201:T15)
            n116 = Unbundle By Name(w201) -> ("Distance (ft)"=w197:dbl)
            n117 = Subtract(x=w196, y=w197) -> (x-y=w199:dbl)
            n118 = global read "Autonomous Global Data.vi" "D1"() -> (w188:dbl)
            n119 = Equal To 0?(x=w197) -> (x = 0?=w195:bool)
            n120 = Equal To 0?(x=w196) -> (x = 0?=w194:bool)
            n121 = Less Than 0?(x=w188) -> (x < 0?=w205:bool)
            n122 = global read "Autonomous Global Data.vi" "R1"() -> (w189:dbl)
            n123 = Or(x=w195, y=w194) -> (x .or. y?=w192:bool)
            n124 = case shown="False" w205 {
              tunnel: w188 -> [w209 w212]
              tunnel: w199 -> [w208 w211]
              tunnel: [w207 w210] -> w198
              frame False {
                n125 = Less Or Equal?(x=w209, y=w208) -> (x <= y?=w207:bool)
              }
              frame True {
                n126 = Greater Or Equal?(x=w212, y=w211) -> (x >= y?=w210:bool)
              }
            }
            n127 = call-poly <vilib>:"WPI_RobotDriveHolonomicDrive.vi"("Rotation"=0.0, "Y"=w189, "X"=0.0, "RobotDriveDevRef"=w190) -> ("RobotDriveDevRef"=w202:T5)  [unwired: 5 in, 2 out]
            n128 = Or(x=w198, y=w192) -> (x .or. y?=w193:bool)
            n129 = Wait (ms)(milliseconds to wait=u32 50) -> ()  [unwired: 1 out]
          }
        }
        frame #1 {
          w217 = 0.0 ("X")
          # "Stop motors"
          n130 = case shown="True" w213 {
            frame False {
              n131 = global read "Robot Global Data.vi" "Frount of  3 Pointer"() -> (w219:dbl)
              n132 = global write "Robot Global Data.vi" "Shooter motor Speed"(w219) -> ()
            }
            frame True {
              n133 = global read "Robot Global Data.vi" "Frount of 2  Pointer"() -> (w220:dbl)
              n134 = global write "Robot Global Data.vi" "Shooter motor Speed"(w220) -> ()
            }
          }
          n135 = call-poly <vilib>:"WPI_RobotDriveHolonomicDrive.vi"("Rotation"=0.0, "Y"=w217, "X"=w217, "RobotDriveDevRef"=w216) -> ("RobotDriveDevRef"=w214:T5)  [unwired: 5 in, 2 out]
          n136 = Wait Until Next ms Multiple(millisecond multiple=u32 500) -> ()  [unwired: 1 out]
        }
        frame #2 {
          # "Shoot Ball 1"
          # "wait .2 sec"
          n137 = global write "Robot Global Data.vi" "Shooter"(TRUE ("Shooter")) -> ()
          n138 = Wait Until Next ms Multiple(millisecond multiple=u32 200) -> ()  [unwired: 1 out]
        }
        frame #3 {
          # "wait 3 sec."
          n139 = global write "Robot Global Data.vi" "Shooter"(FALSE ("Shooter")) -> ()
          n140 = Wait Until Next ms Multiple(millisecond multiple=u32 3000) -> ()  [unwired: 1 out]
        }
        frame #4 {
          # "Shoot Ball 2"
          # "wait .2 sec"
          n141 = global write "Robot Global Data.vi" "Shooter"(TRUE ("Shooter")) -> ()
          n142 = Wait Until Next ms Multiple(millisecond multiple=u32 200) -> ()  [unwired: 1 out]
        }
        frame #5 {
          # "wait 3 sec."
          n143 = global write "Robot Global Data.vi" "Shooter"(FALSE ("Shooter")) -> ()
          n144 = Wait Until Next ms Multiple(millisecond multiple=u32 3000) -> ()  [unwired: 1 out]
        }
      }
      n145 = call <vilib>:"WPI_RobotDriveSafetyConfig.vi"("mode"=WPI_SafetyOutputConfigMenu."Disable", "RobotDriveDevRef"=w171) -> ()  [unwired: 8 in, 2 out]
    }
    frame 5 {
      n146 = flat-sequence {
        frame #0 {
          n147 = Wait Until Next ms Multiple(millisecond multiple=u32 250) -> ()  [unwired: 1 out]
        }
        frame #1 {
          # "Stop motors"
          n148 = global read "Robot Global Data.vi" "Key of  3 Pointer"() -> (w234:dbl)
          n149 = global write "Robot Global Data.vi" "Shooter motor Speed"(w234) -> ()
        }
        frame #2 {
          # "Shoot Ball 1"
          # "wait .2 sec"
          n150 = global write "Robot Global Data.vi" "Shooter"(TRUE ("Shooter")) -> ()
          n151 = Wait Until Next ms Multiple(millisecond multiple=u32 500) -> ()  [unwired: 1 out]
        }
        frame #3 {
          # "wait 3 sec."
          n152 = global write "Robot Global Data.vi" "Shooter"(FALSE ("Shooter")) -> ()
          n153 = Wait Until Next ms Multiple(millisecond multiple=u32 4000) -> ()  [unwired: 1 out]
        }
        frame #4 {
          # "Shoot Ball 2"
          # "wait .2 sec"
          n154 = global write "Robot Global Data.vi" "Shooter"(TRUE ("Shooter")) -> ()
          n155 = Wait Until Next ms Multiple(millisecond multiple=u32 500) -> ()  [unwired: 1 out]
        }
        frame #5 {
          # "wait 3 sec."
          n156 = global write "Robot Global Data.vi" "Shooter"(FALSE ("Shooter")) -> ()
          n157 = Wait Until Next ms Multiple(millisecond multiple=u32 4000) -> ()  [unwired: 1 out]
        }
      }
    }
    frame 6 {
      # "2/3 Point auto"
      # "Autonomous of Six"
      n158 = flat-sequence {
        tunnel: [w262] -> w253
        tunnel: [w261] -> w252
        tunnel: w244 -> [w256]
        tunnel: [w254] -> w243
        tunnel: w253 -> [w300]
        tunnel: w252 -> [w298]
        tunnel: [w297] -> w250
        tunnel: w245 -> [w296]
        tunnel: w243 -> [w295]
        tunnel: [w312] -> w251
        tunnel: w250 -> [w312]
        tunnel: w251 -> [w315]
        tunnel: [w315] -> w248
        tunnel: [w318] -> w249
        tunnel: w248 -> [w318]
        tunnel: w249 -> [w321]
        tunnel: [w321] -> w247
        frame #0 {
          # "Use three point from key"
          n159 = global read "Robot Global Data.vi" "Target Info"() -> (w265:T14)
          n160 = Index Array(array=w265, index=0) -> (element=w264:T15)
          n161 = Unbundle By Name(w264) -> ("Distance (ft)"=w263:dbl)
          n162 = call <vilib>:"WPI_RobotDriveRefNum Registry Get.vi"("refnum name"="d_motors") -> ("RobotDriveDevRef"=w259:T5)  [unwired: 1 in, 9 out]
          n163 = call <vilib>:"WPI_RobotDriveSafetyConfig.vi"("mode"=WPI_SafetyOutputConfigMenu."Disable", "RobotDriveDevRef"=w259) -> ("RobotDriveDevRef"=w257:T5)  [unwired: 8 in, 1 out]
          n164 = while {
            tunnel: w263 -> [w270]
            tunnel: [w284] -> w262
            tunnel: [w275] -> w261
            tunnel: w257 -> [w276]
            tunnel: w256 -> [w269]
            shift-right: [w273] -> _
            shift-left: 0.0 ("R1") -> [w274]
            tunnel: [w267] -> w254
            stop <- w279 stop-if-true
            # "Rate to Target"
            # "Distance to trave"
            # "note:Key is located 144 in. from the Alliance Wal\nFender is 38-3/4 in. deepl"
            # "Drive for"
            # "Feet"
            # "RUN"
            # "Case handles negative or positive setpoints"
            # "End?"
            # "Stop when one side reaches the setpoint"
            n165 = global read "Robot Global Data.vi" "Target Info"() -> (w277:T14)
            n166 = Index Array(array=w277, index=0) -> (element=w283:T15)
            n167 = Unbundle By Name(w283) -> ("Distance (ft)"=w271:dbl)
            n168 = Equal To 0?(x=w271) -> (x = 0?=w280:bool)
            n169 = Equal To 0?(x=w270) -> (x = 0?=w268:bool)
            n170 = Or(x=w280, y=w268) -> (x .or. y?=w278:bool)
            n171 = global read "Autonomous Global Data.vi" "D1"() -> (w272:dbl)
            n172 = Less Than 0?(x=w272) -> (x < 0?=w287:bool)
            n173 = case shown="True" w287 {
              tunnel: w272 -> [w291 w294]
              tunnel: w271 -> [w290 w293]
              tunnel: [w289 w292] -> w281
              frame False {
                n174 = Greater Or Equal?(x=w291, y=w290) -> (x >= y?=w289:bool)
              }
              frame True {
                n175 = Less Or Equal?(x=w294, y=w293) -> (x <= y?=w292:bool)
              }
            }
            n176 = call-poly <vilib>:"WPI_RobotDriveHolonomicDrive.vi"("Rotation"=0.0, "Y"=w274, "X"=0.0, "RobotDriveDevRef"=w276) -> ("RobotDriveDevRef"=w284:T5)  [unwired: 5 in, 2 out]
            n177 = Or(x=w278, y=w269) -> (x .or. y?=w275:bool)
            n178 = Or(x=w281, y=w275) -> (x .or. y?=w279:bool)
            n179 = Or(x=w268, y=w269) -> (x .or. y?=w267:bool)
            n180 = global read "Autonomous Global Data.vi" "R1"() -> (w273:dbl)
            n181 = Wait (ms)(milliseconds to wait=u32 50) -> ()  [unwired: 1 out]
          }
        }
        frame #1 {
          w301 = 0.0 ("X")
          # "True - Top Hoop\nFalse -  Mid Hoop"
          # "Stop motors"
          n182 = case shown="True" w295 {
            tunnel: w298 -> [w304 _]
            tunnel: w296 -> [w303 _]
            frame False {
              n183 = case shown="False" w303 {
                tunnel: w304 -> [w305 w308]
                frame False {
                  n184 = case shown="True" w305 {
                    frame False {
                      n185 = global read "Robot Global Data.vi" "Frount of 2  Pointer"() -> (w306:dbl)
                      n186 = global write "Robot Global Data.vi" "Shooter motor Speed"(w306) -> ()
                    }
                    frame True {
                      n187 = global read "Robot Global Data.vi" "Frount of  3 Pointer"() -> (w307:dbl)
                      n188 = global write "Robot Global Data.vi" "Shooter motor Speed"(w307) -> ()
                    }
                  }
                }
                frame True {
                  n189 = case shown="True" w308 {
                    frame False {
                      n190 = global read "Robot Global Data.vi" "Frount of  3 Pointer"() -> (w309:dbl)
                      n191 = global write "Robot Global Data.vi" "Shooter motor Speed"(w309) -> ()
                    }
                    frame True {
                      n192 = global read "Robot Global Data.vi" "Frount of  3 Pointer"() -> (w310:dbl)
                      n193 = global write "Robot Global Data.vi" "Shooter motor Speed"(w310) -> ()
                    }
                  }
                }
              }
            }
            frame True {
              n194 = global read "Robot Global Data.vi" "Key of  3 Pointer"() -> (w311:dbl)
              n195 = global write "Robot Global Data.vi" "Shooter motor Speed"(w311) -> ()
            }
          }
          n196 = call-poly <vilib>:"WPI_RobotDriveHolonomicDrive.vi"("Rotation"=0.0, "Y"=w301, "X"=w301, "RobotDriveDevRef"=w300) -> ("RobotDriveDevRef"=w297:T5)  [unwired: 5 in, 2 out]
          n197 = Wait Until Next ms Multiple(millisecond multiple=u32 500) -> ()  [unwired: 1 out]
        }
        frame #2 {
          # "Shoot Ball 1"
          # "wait .2 sec"
          n198 = global write "Robot Global Data.vi" "Shooter"(TRUE ("Shooter")) -> ()
          n199 = Wait Until Next ms Multiple(millisecond multiple=u32 200) -> ()  [unwired: 1 out]
        }
        frame #3 {
          # "wait 3 sec."
          n200 = global write "Robot Global Data.vi" "Shooter"(FALSE ("Shooter")) -> ()
          n201 = Wait Until Next ms Multiple(millisecond multiple=u32 3000) -> ()  [unwired: 1 out]
        }
        frame #4 {
          # "Shoot Ball 2"
          # "wait .2 sec"
          n202 = global write "Robot Global Data.vi" "Shooter"(TRUE ("Shooter")) -> ()
          n203 = Wait Until Next ms Multiple(millisecond multiple=u32 200) -> ()  [unwired: 1 out]
        }
        frame #5 {
          # "wait 3 sec."
          n204 = global write "Robot Global Data.vi" "Shooter"(FALSE ("Shooter")) -> ()
          n205 = Wait Until Next ms Multiple(millisecond multiple=u32 3000) -> ()  [unwired: 1 out]
        }
      }
      n206 = call <vilib>:"WPI_RobotDriveSafetyConfig.vi"("mode"=WPI_SafetyOutputConfigMenu."Disable", "RobotDriveDevRef"=w247) -> ()  [unwired: 8 in, 2 out]
    }
    frame 7 {
      n207 = flat-sequence {
        tunnel: [w344] -> w336
        tunnel: w331 -> [w345]
        tunnel: [w343] -> w329
        tunnel: [w342] -> w328
        tunnel: "time" -> [_]
        tunnel: w336 -> [w370]
        tunnel: [w368] -> w335
        tunnel: w330 -> [w366]
        tunnel: w329 -> [w367]
        tunnel: w328 -> [w365]
        tunnel: [w364] -> w327
        tunnel: [w383] -> w334
        tunnel: w335 -> [w383]
        tunnel: w327 -> [w382]
        tunnel: [w382] -> w325
        tunnel: w334 -> [w387]
        tunnel: [w387] -> w333
        tunnel: [w386] -> w326
        tunnel: w325 -> [w386]
        tunnel: [w391] -> w332
        tunnel: w333 -> [w391]
        tunnel: w326 -> [w390]
        tunnel: w332 -> [w394]
        tunnel: [w394] -> _
        frame #0 {
          # "Use three point from key"
          n208 = global read "Autonomous Global Data.vi" "D3"() -> (w337:dbl)
          n209 = call <vilib>:"WPI_RobotDriveRefNum Registry Get.vi"("refnum name"="d_motors") -> ("RobotDriveDevRef"=w349:T5)  [unwired: 1 in, 9 out]
          n210 = call <vilib>:"WPI_RobotDriveSafetyConfig.vi"("mode"=WPI_SafetyOutputConfigMenu."Disable", "RobotDriveDevRef"=w349) -> ("RobotDriveDevRef"=w347:T5)  [unwired: 8 in, 1 out]
          n211 = Multiply(x=w337, y=1000.0) -> (x*y=w341:dbl)
          n212 = Divide(x=w341, y=50.0) -> (x/y=w339:dbl)
          n213 = while {
            tunnel: w347 -> [w357]
            tunnel: w339 -> [w361]
            tunnel: [w358] -> w344
            tunnel: w345 -> [w360]
            tunnel: [w360] -> w343
            tunnel: [w359] -> w342
            shift-right: [w354] -> _
            shift-left: 0 -> [w353]
            i -> [w354]
            stop <- w359 stop-if-true
            # "Drive?"
            n214 = Increment(x=w353) -> (x+1=w363:i32)
            n215 = Greater Or Equal?(x=w363, y=w361) -> (x >= y?=w362:bool)
            n216 = Wait Until Next ms Multiple(millisecond multiple=u32 50) -> ()  [unwired: 1 out]
            n217 = call-poly <vilib>:"WPI_RobotDriveHolonomicDrive.vi"("Rotation"=0.0, "Y"=-0.5 ("Scale (%)"), "X"=0.0, "RobotDriveDevRef"=w357) -> ("RobotDriveDevRef"=w358:T5)  [unwired: 5 in, 2 out]
            n218 = Or(x=w362, y=w360) -> (x .or. y?=w359:bool)
          }
        }
        frame #1 {
          w371 = 0.0 ("X")
          # "True - Top Hoop\nFalse -  Mid Hoop"
          # "Stop motors"
          n219 = case shown="False" w367 {
            tunnel: w366 -> [w375 _]
            tunnel: w365 -> [w374 _]
            tunnel: [w373 w381] -> w364
            frame False {
              n220 = case shown="True" w374 {
                tunnel: w375 -> [_ w378]
                tunnel: [w376 w377] -> w373
                frame False {
                  n221 = global read "Robot Global Data.vi" "Frount of  3 Pointer"() -> (w376:dbl)
                  n222 = global write "Robot Global Data.vi" "Shooter motor Speed"(w376) -> ()
                }
                frame True {
                  n223 = case shown="True" w378 {
                    tunnel: [w379 w380] -> w377
                    frame False {
                      n224 = global read "Robot Global Data.vi" "Frount of  3 Pointer"() -> (w379:dbl)
                      n225 = global write "Robot Global Data.vi" "Shooter motor Speed"(w379) -> ()
                    }
                    frame True {
                      n226 = global read "Robot Global Data.vi" "Frount of 2  Pointer"() -> (w380:dbl)
                      n227 = global write "Robot Global Data.vi" "Shooter motor Speed"(w380) -> ()
                    }
                  }
                }
              }
            }
            frame True {
              n228 = global read "Robot Global Data.vi" "Key of  3 Pointer"() -> (w381:dbl)
              n229 = global write "Robot Global Data.vi" "Shooter motor Speed"(w381) -> ()
            }
          }
          n230 = call-poly <vilib>:"WPI_RobotDriveHolonomicDrive.vi"("Rotation"=0.0, "Y"=w371, "X"=w371, "RobotDriveDevRef"=w370) -> ("RobotDriveDevRef"=w368:T5)  [unwired: 5 in, 2 out]
          n231 = Wait Until Next ms Multiple(millisecond multiple=u32 500) -> ()  [unwired: 1 out]
        }
        frame #2 {
          # "Shoot Ball 1"
          # "wait .2 sec"
          n232 = global write "Robot Global Data.vi" "Shooter motor Speed"(w382) -> ()
          n233 = global write "Robot Global Data.vi" "Shooter"(TRUE ("Shooter")) -> ()
          n234 = Wait Until Next ms Multiple(millisecond multiple=u32 200) -> ()  [unwired: 1 out]
        }
        frame #3 {
          # "wait 3 sec."
          n235 = global write "Robot Global Data.vi" "Shooter"(FALSE ("Shooter")) -> ()
          n236 = Wait Until Next ms Multiple(millisecond multiple=u32 3000) -> ()  [unwired: 1 out]
        }
        frame #4 {
          # "Shoot Ball 2"
          # "wait .2 sec"
          n237 = global write "Robot Global Data.vi" "Shooter motor Speed"(w390) -> ()
          n238 = global write "Robot Global Data.vi" "Shooter"(TRUE ("Shooter")) -> ()
          n239 = Wait Until Next ms Multiple(millisecond multiple=u32 200) -> ()  [unwired: 1 out]
        }
        frame #5 {
          # "wait 3 sec."
          n240 = Wait Until Next ms Multiple(millisecond multiple=u32 3000) -> ()  [unwired: 1 out]
          n241 = global write "Robot Global Data.vi" "Shooter"(FALSE ("Shooter")) -> ()
        }
      }
    }
    frame 8 {
      n242 = call <vilib>:"WPI_MotorControlRefNum Registry Get.vi"("refnum name"="Sweeper Drive Motor ") -> ("MotorControlDevRef"=w397:T6)  [unwired: 9 in, 1 out]
      n243 = call <vilib>:"WPI_MotorControlRefNum Registry Get.vi"("refnum name"="Belt Drive Motor ") -> ("MotorControlDevRef"=w398:T6)  [unwired: 9 in, 1 out]
      n244 = flat-sequence {
        tunnel: [w410] -> w406
        tunnel: w397 -> [w410]
        tunnel: w398 -> [w409]
        tunnel: [w409] -> w405
        tunnel: w406 -> [w415]
        tunnel: w405 -> [w414]
        tunnel: [w413] -> w402
        tunnel: [w412] -> w400
        tunnel: w402 -> [w428]
        tunnel: [w431] -> w401
        tunnel: w400 -> [w429]
        tunnel: [w430] -> w399
        tunnel: w401 -> [w435]
        tunnel: [w432] -> w404
        tunnel: w399 -> [w434]
        tunnel: [w433] -> w403
        tunnel: w404 -> [w447]
        tunnel: w403 -> [w448]
        frame #0 {
          n245 = global read "Autonomous Global Data.vi" "COV Waito"() -> (w411:dbl)
          n246 = Wait Until Next ms Multiple(millisecond multiple=w411) -> ()  [unwired: 1 out]
        }
        frame #1 {
          n247 = while {
            tunnel: w415 -> [w425]
            tunnel: w414 -> [w424]
            tunnel: [w423] -> w413
            tunnel: [w422] -> w412
            i -> [w419]
            stop <- w418 stop-if-true
            n248 = global read "Autonomous Global Data.vi" "COV Speede"() -> (w421:dbl)
            n249 = Negate(x=w421) -> (-x=w416:dbl)
            n250 = Increment(x=w419) -> (x+1=w420:i32)
            n251 = call <vilib>:"WPI_MotorControlSetOutput.vi"("Output"=w421, "MotorControlDevRef"=w424) -> ("MotorControlDevRef"=w423:T6)  [unwired: 7 in, 2 out]
            n252 = call <vilib>:"WPI_MotorControlSetOutput.vi"("Output"=w416, "MotorControlDevRef"=w425) -> ("MotorControlDevRef"=w422:T6)  [unwired: 7 in, 2 out]
            n253 = Greater Or Equal?(x=w420, y=u32 500 ("millisecond multiple")) -> (x >= y?=w418:bool)
          }
        }
        frame #2 {
          w427 = 0
          n254 = Wait Until Next ms Multiple(millisecond multiple=u32 1000) -> ()  [unwired: 1 out]
          n255 = call <vilib>:"WPI_MotorControlSetOutput.vi"("Output"=w427, "MotorControlDevRef"=w428) -> ("MotorControlDevRef"=w431:T6)  [unwired: 7 in, 2 out]
          n256 = call <vilib>:"WPI_MotorControlSetOutput.vi"("Output"=w427, "MotorControlDevRef"=w429) -> ("MotorControlDevRef"=w430:T6)  [unwired: 7 in, 2 out]
        }
        frame #3 {
          n257 = while {
            tunnel: w434 -> [w445]
            tunnel: w435 -> [w444]
            tunnel: [w443] -> w432
            tunnel: [w442] -> w433
            i -> [w439]
            stop <- w438 stop-if-true
            n258 = global read "Autonomous Global Data.vi" "COV Speede"() -> (w441:dbl)
            n259 = Negate(x=w441) -> (-x=w436:dbl)
            n260 = Increment(x=w439) -> (x+1=w440:i32)
            n261 = call <vilib>:"WPI_MotorControlSetOutput.vi"("Output"=w441, "MotorControlDevRef"=w444) -> ("MotorControlDevRef"=w443:T6)  [unwired: 7 in, 2 out]
            n262 = call <vilib>:"WPI_MotorControlSetOutput.vi"("Output"=w436, "MotorControlDevRef"=w445) -> ("MotorControlDevRef"=w442:T6)  [unwired: 7 in, 2 out]
            n263 = Greater Or Equal?(x=w440, y=u32 500 ("millisecond multiple")) -> (x >= y?=w438:bool)
          }
        }
        frame #4 {
          w446 = 0.0 ("Output")
          n264 = call <vilib>:"WPI_MotorControlSetOutput.vi"("Output"=w446, "MotorControlDevRef"=w447) -> ()  [unwired: 7 in, 3 out]
          n265 = call <vilib>:"WPI_MotorControlSetOutput.vi"("Output"=w446, "MotorControlDevRef"=w448) -> ()  [unwired: 7 in, 3 out]
        }
      }
    }
  }
  n266 = global write "Robot Global Data.vi" "LED toggle rate (ms)"(u32 500 ("LED ms toggle rate")) -> ()
